vi "Pulse Timer.vi"(7 "Initialize":bool, 8 "Error In":errorcluster, 10 "Off Time":u32=10, 11 "On Time":u32=1) -> (0 "Error Out":errorcluster, 3 "Boolean Out":bool)   [LabVIEW 2014]
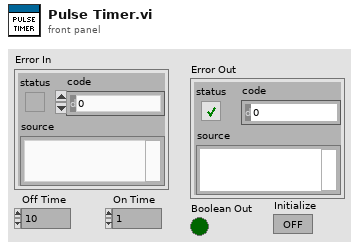
[diagram p1: front panel]
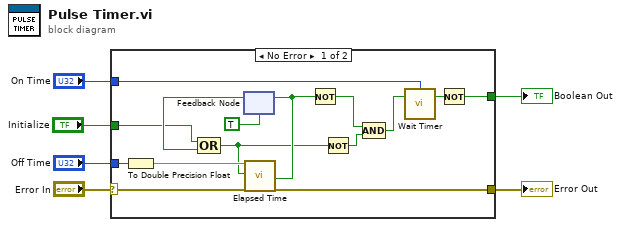
[diagram p0: block diagram]
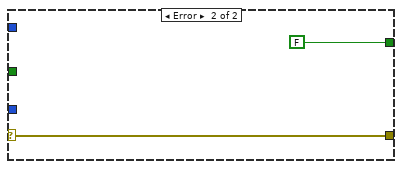
[diagram p2: hidden frame]
diagram:
  n1 = case shown="No Error" "Error In" {
    selector: "Error In" -> [w18 w23]
    tunnel: [w17 w23] -> w5
    tunnel: "Off Time" -> [w16 _]
    tunnel: "On Time" -> [w15 _]
    tunnel: [w7 FALSE] -> w2
    tunnel: "Initialize" -> [w12 _]
    frame No Error {
      n2 = To Double Precision Float(number=w16) -> (double precision float=w14:dbl)
      n3 = feedback #1(TRUE ("Boolean Out")) -> (w13:bool)
      n4 = Compound Arithmetic op=OR(w12, w13) -> (w9:bool)
      n5 = call "Elapsed Time"("Time Target (s)"=w14, "Reset"=w9, "error in (no error)"=w18) -> ("Time has Elapsed"=w19:bool, "error out"=w17:errorcluster)  [unwired: 9 in, 6 out]
      n6 = feedback-in #1(w19) -> ()
      n7 = Not(x=w19) -> (.not. x?=w11:bool)
      n8 = Not(x=w9) -> (.not. x?=w8:bool)
      n9 = Compound Arithmetic op=AND(w11, w8) -> (w10:bool)
      n10 = call "Wait Timer.vi"("Boolean In"=w10, "Timer"=w15) -> ("Boolean Out"=w21:bool)  [unwired: 3 in]
      n11 = Not(x=w21) -> (.not. x?=w7:bool)
    }
    frame Error {
    }
  }
  "Error Out" <- w5
  "Boolean Out" <- w2
